vi "Data-log-write-file.vi"(7 "Interval":dbl=0.01, 8 "error in (no error)":errorcluster, 10 "Data cluster in":cluster{"Plant 2":T1, "Plant 1":T1}) -> (0 "error out":errorcluster, 2 "new file path":path)   [LabVIEW 2016]
uses:
  Plant-data.ctl
  <vilib>/Utility/file.llb/Write Delimited Spreadsheet (DBL).vi
panel:
  out "data array":dbl[][](array[numeric])
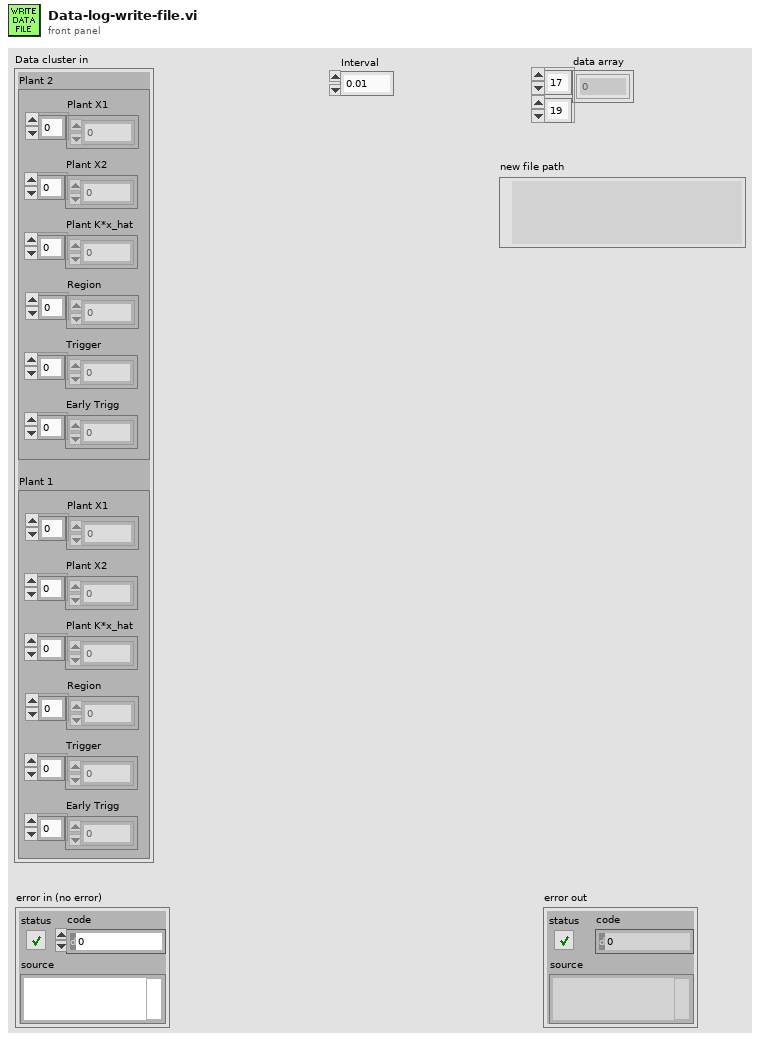
[diagram p1: front panel]
types:
  T1 = typedef "Plant-data.ctl" = cluster{"Plant X1 ":dbl[], "Plant X2":dbl[], "Plant K*x_hat":dbl[], "Region":i32[], "Trigger":i32[], "Early Trigg":i32[]}
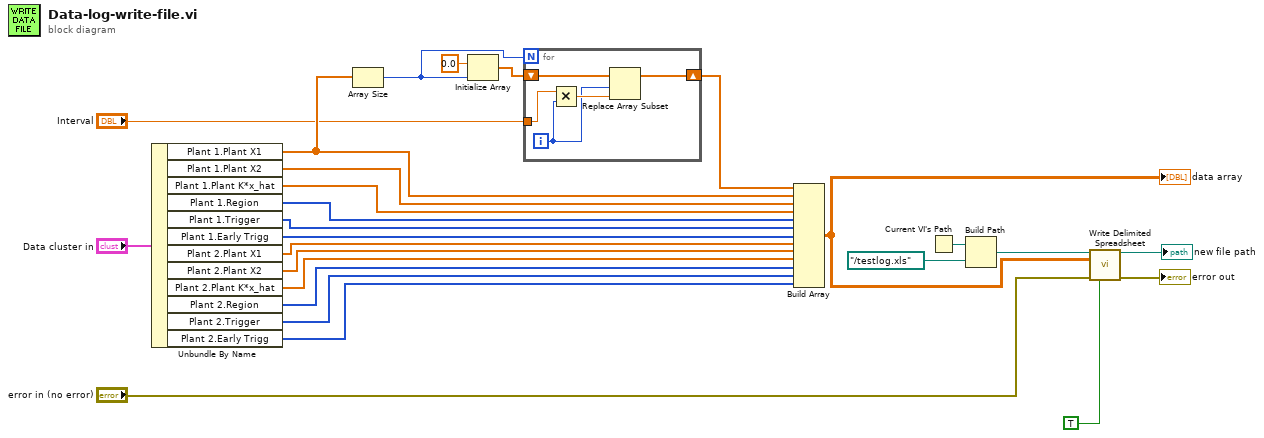
[diagram p0: block diagram]
diagram:
  n1 = Unbundle By Name("Data cluster in") -> ("Plant 1.Plant X1"=w20:dbl[], "Plant 1.Plant X2"=w25:dbl[], "Plant 1.Plant K*x_hat"=w24:dbl[], "Plant 1.Region"=w23:i32[], "Plant 1.Trigger"=w22:i32[], "Plant 1.Early Trigg"=w21:i32[], "Plant 2.Plant X1"=w8:dbl[], "Plant 2.Plant X2"=w7:dbl[], "Plant 2.Plant K*x_hat"=w6:dbl[], "Plant 2.Region"=w5:i32[], "Plant 2.Trigger"=w4:i32[], "Plant 2.Early Trigg"=w3:i32[])
  n2 = Array Size(array=w20) -> (size(s)=w15:i32)
  n3 = Initialize Array(0.0 ("element"), w15) -> (w16:dbl[])
  n4 = for {
    N: w15 -> [_]
    tunnel: "Interval" -> [w29]
    shift-right: [w28] -> w17
    shift-left: w16 -> [w31]
    i -> [w27]
    n5 = Multiply(x=w29, y=w27) -> (x*y=w30:dbl)
    n6 = Replace Array Subset(array=w31, new element=w30, index=w27) -> (w28:dbl[])
  }
  n7 = Build Array(w17, w20, w25, w24, w23, w22, w21, w8, w7, w6, w5, w4, w3) -> (w14:dbl[][])
  "data array" <- w14
  n8 = Current VI's Path() -> (path=w12:path)
  n9 = Build Path(base path=w12, name or relative path=path "../testlog.xls" ("file path (dialog if empty)")) -> (appended path=w2:path)
  n10 = call-poly <vilib>:"Write Delimited Spreadsheet.vi"("file path (dialog if empty)"=w2, "2D data"=w14, "error in (no error)"="error in (no error)", "transpose? (no:F)"=TRUE) -> ("new file path (Not A Path if cancelled)"=→"new file path":path, "error out"=→"error out":errorcluster)  [unwired: 10 in]
